vi "ao_ai_dmm_amp_test.vi"() -> ()   [LabVIEW 2020]
uses:
  Realization/PIPX40 Matrix/PIPX40 Matrix.lvclass
  Realization/NI Analog Input/NI Analog Input.lvclass
  Realization/NI DAQmx Base/TypeDefs/Channel Config.ctl
  Realization/NI Analog Output/TypeDefs/Timing Config.ctl
  Realization/NI Analog Output/NI Analog Output.lvclass
  Realization/PIPX40 Relay/PIPX40 Relay.lvclass
  Realization/NI DMM/NI DMM.lvclass
  Realization/PI650 VoltageAmp/PI650 VoltageAmp.lvclass
  Realization/PI650 VoltageAmp/TypeDefs/Channel gain.ctl
  Realization/PI650 VoltageAmp/TypeDefs/Channel DC offset.ctl
  Realization/NI DMM/TypeDefs/DMM waveform settings.ctl
  <instrlib>/niDMM/nidmm.llb/niDMM Waveform Function.ctl
  <instrlib>/niDMM/nidmm.llb/niDMM Function.ctl
panel:
  out "Amp Info":variant
  out "DMM":waveform(dbl)(graph)
  out "DMM Info":variant
  out "AI":waveform(dbl)[](graph)
  out "relay info":variant
  out "AO Info":variant
  out "AI infos":variant[](array[variant])
  out "Mx infos":variant[](array[variant])
  out "error out":errorcluster
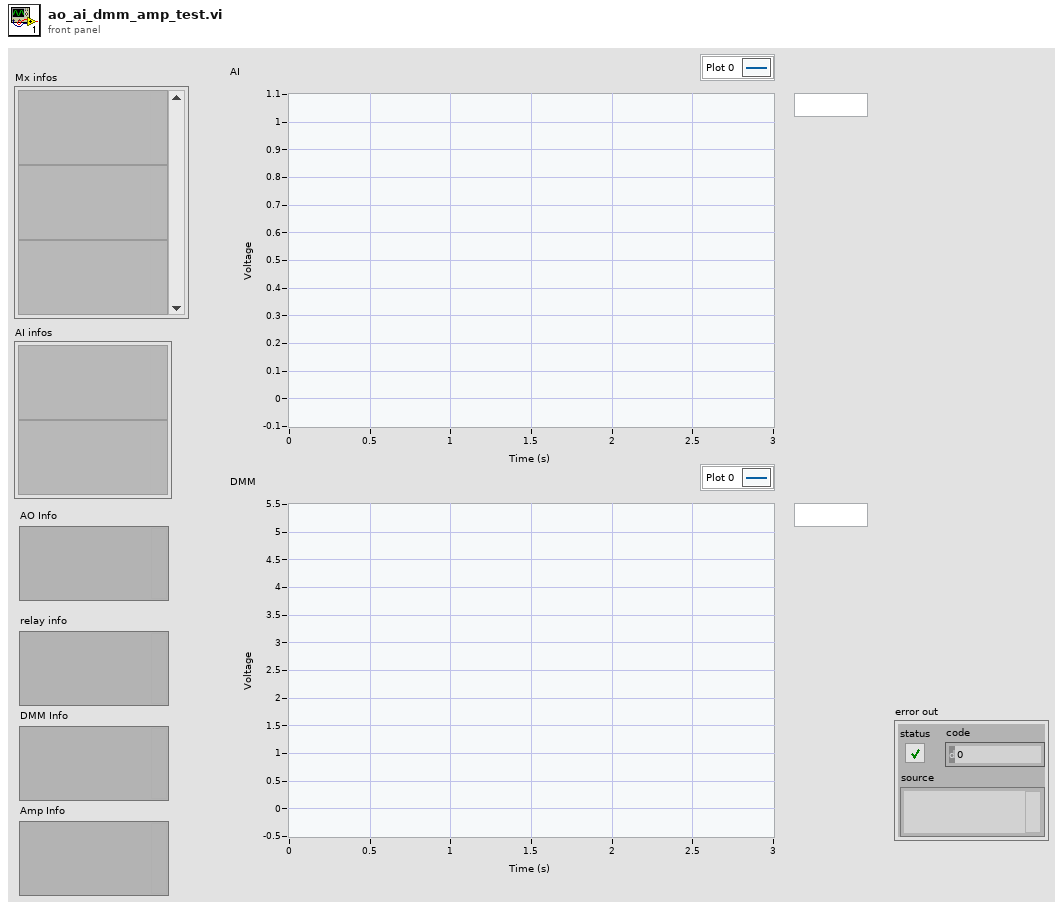
[diagram p1: front panel]
types:
  T1 = typedef "Channel gain.ctl" = cluster{"Channel (CH1)":u32, "Gain (x1)":u32}
  T2 = typedef "Channel Config.ctl" = cluster{"channels":string, "maximum value":dbl, "minimum value":dbl, "output terminal configuration":i32, "units":i32}
  T3 = map{string, refnum<class "NI Analog Input.lvclass">}
  T4 = map{string, refnum<class "PIPX40 Matrix.lvclass">}
  T5 = typedef "Timing Config.ctl" = cluster{"sample mode":i32, "samples per channel":i32, "rate":dbl, "source":string, "active edge":i32}
  T6 = typedef "Rendezvous RefNum" = refnum<k1>
  T7 = typedef "Channel DC offset.ctl" = cluster{"Channel (CH1)":u32, "Offset (128)":u32}
  T8 = typedef "niDMM Function.ctl" = enum16{"DC Volts", "AC Volts", "DC Current", "AC Current", "2-wire Resistance", "4-wire Resistance", "Diode", "Frequency", "Period", "AC Volts DC Coupled", "Capacitance", "Inductance", "Temperature"}
  T9 = cluster{"Function":T8, "Resolution":dbl, "Range":dbl}
  T10 = typedef "DMM waveform settings.ctl" = cluster{"Waveform Points":i32, "Function":T11, "Rate":dbl, "Range":dbl, "Settle Time":dbl}
  T11 = typedef "niDMM Waveform Function.ctl" = i32
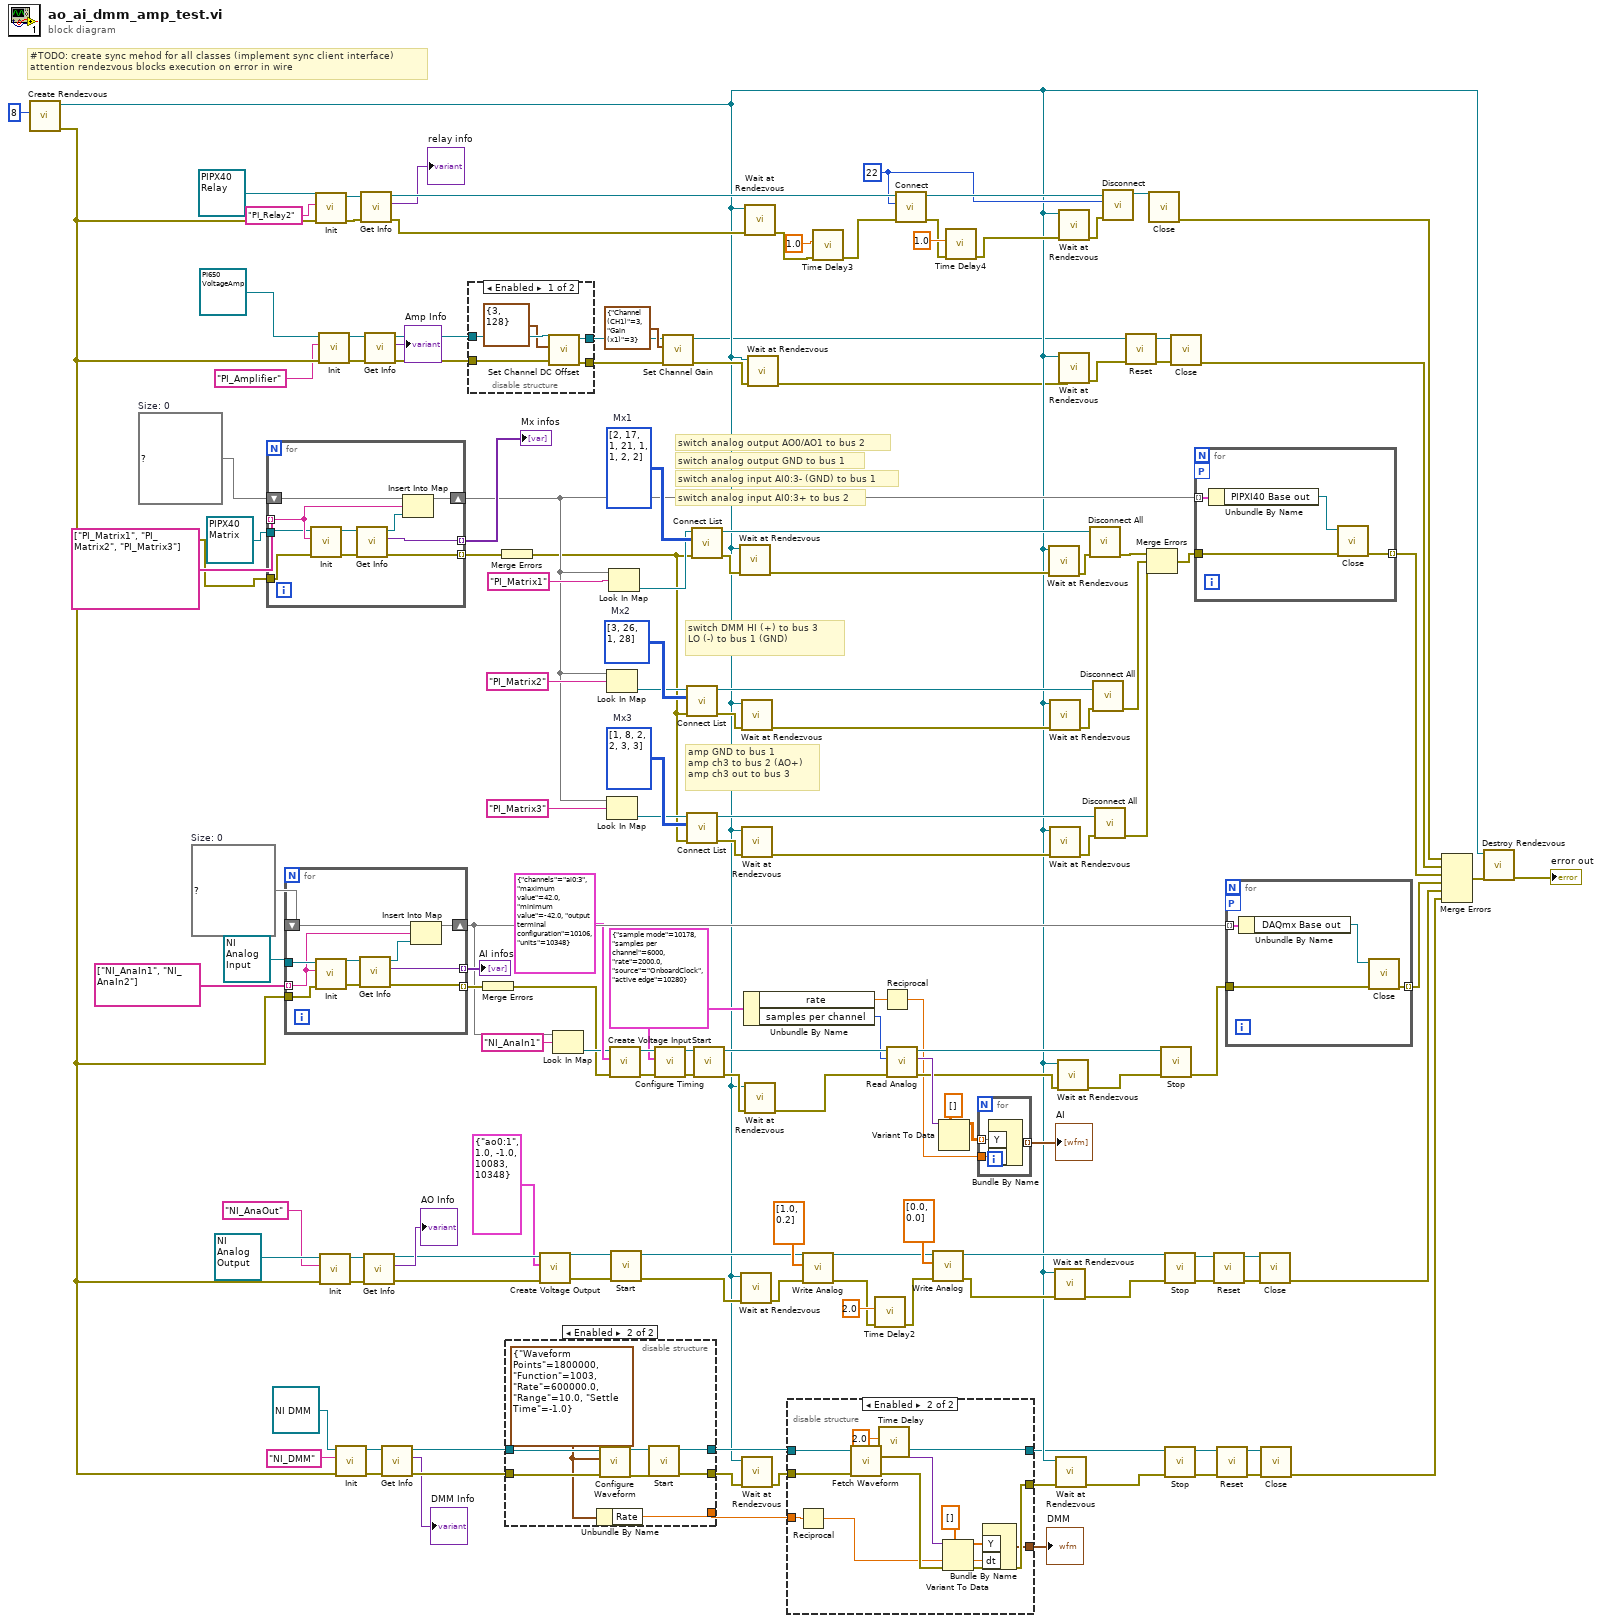
[diagram p0: block diagram]
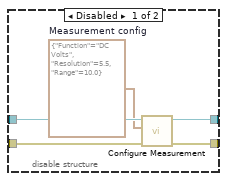
[diagram p3: hidden frame]
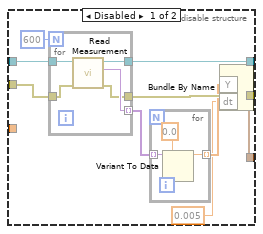
[diagram p4: hidden frame]
diagram:
  w18 = i32[][] [[1, 8], [2, 2], [3, 3]]  # Mx3
  w69 = 22
  w120 = T3 {}  # Size: 0
  w126 = T4 {}  # Size: 0
  w48 = T5 {"sample mode"=10178, "samples per channel"=6000, "rate"=2000.0, "source"="OnboardClock", "active edge"=10280}
  w144 = i32[][] [[3, 26], [1, 28]]  # Mx2
  w146 = i32[][] [[2, 17], [1, 21], [1, 1], [2, 2]]  # Mx1
  # "amp GND to bus 1\namp ch3 to bus 2 (AO+) \namp ch3 out to bus 3"
  # "switch analog input AI0:3+ to bus 2"
  # "switch analog input AI0:3- (GND) to bus 1"
  # "switch analog output GND to bus 1"
  # "switch analog output AO0/AO1 to bus 2"
  # "switch DMM HI (+) to bus 3 \nLO (-) to bus 1 (GND)"
  # "#TODO: create sync mehod for all classes (implement sync client interface)\nattention rendezvous blocks execution on error in wire"
  n1 = call <vilib>:"Create Rendezvous.vi"("size (2)"=8) -> ("error out"=w37:errorcluster, "rendezvous"=w10:T6)  [unwired: 4 in, 1 out]
  n2 = for {
    tunnel: string[] ["PI_Matrix1", "PI_Matrix2", "PI_Matrix3"] -> [w157] mode=indexing
    tunnel: [w160] -> w150 mode=indexing
    tunnel: [w159] -> w148 mode=indexing
    shift-right: [w158] -> w12
    shift-left: w126 -> [w155]
    tunnel: refnum<class "PIPX40 Matrix.lvclass"> refnum ("PIPXI40 Matrix in") -> [w153]
    tunnel: w37 -> [w152]
    n3 = call-dynamic "Init.vi"("error in (no error)"=w152, "Params"=w157, "PIPXI40 Base in"=w153) -> ("error out"=w161:errorcluster, "PIPXI40 Base out"=w156:refnum<class "PIPX40 Matrix.lvclass">)  [unwired: 7 in]
    n4 = call-dynamic "Get Info.vi"("error in (no error)"=w161, "PIPXI40 Base in"=w156) -> ("error out"=w160:errorcluster, "Info"=w159:variant, "PIPXI40 Base out"=w154:refnum<class "PIPX40 Matrix.lvclass">)  [unwired: 7 in]
    n5 = Insert Into Map(map in=w155, key=w157, value=w154) -> (map out=w158:T4)  [unwired: 2 out]
  }
  "Mx infos" <- w148
  n6 = for {
    tunnel: string[] ["NI_AnaIn1", "NI_AnaIn2"] -> [w163] mode=indexing
    shift-right: [w171] -> w134
    shift-left: w120 -> [w170]
    tunnel: refnum<class "NI Analog Input.lvclass"> refnum ("NI Analog Input in") -> [w169]
    tunnel: [w165] -> w137 mode=indexing
    tunnel: [w164] -> w136 mode=indexing
    tunnel: w37 -> [w162]
    n7 = call-dynamic "Init.vi"("error in (no error)"=w162, "Params"=w163, "DAQmx Base in"=w169) -> ("error out"=w167:errorcluster, "DAQmx Base out"=w168:refnum<class "NI Analog Input.lvclass">)  [unwired: 7 in]
    n8 = call-dynamic "Get Info.vi"("error in (no error)"=w167, "DAQmx Base in"=w168) -> ("error out"=w164:errorcluster, "Info"=w165:variant, "DAQmx Base out"=w166:refnum<class "NI Analog Input.lvclass">)  [unwired: 7 in]
    n9 = Insert Into Map(map in=w170, key=w163, value=w166) -> (map out=w171:T3)  [unwired: 2 out]
  }
  "AI infos" <- w137
  n10 = call-dynamic "Init.vi"("error in (no error)"=w37, "Params"="PI_Relay2" ("String"), "PIPXI40 Base in"=refnum<class "PIPX40 Relay.lvclass"> refnum ("Pickering.lvlib:PIPX40 Relay.lvclass")) -> ("error out"=w106:errorcluster, "PIPXI40 Base out"=w103:refnum<class "PIPX40 Relay.lvclass">)  [unwired: 7 in]
  n11 = call-dynamic "Init.vi"("error in (no error)"=w37, "Params"="PI_Amplifier" ("String"), "PI650 VoltageAmp in"=refnum<class "PI650 VoltageAmp.lvclass"> refnum) -> ("error out"=w28:errorcluster, "PI650 VoltageAmp out"=w29:refnum<class "PI650 VoltageAmp.lvclass">)  [unwired: 7 in]
  n12 = call-dynamic "Init.vi"("error in (no error)"=w37, "Params"="NI_AnaOut" ("String"), "DAQmx Base in"=refnum<class "NI Analog Output.lvclass"> refnum ("NI DAQmx.lvlib:NI Analog Output.lvclass")) -> ("error out"=w118:errorcluster, "DAQmx Base out"=w119:refnum<class "NI Analog Output.lvclass">)  [unwired: 7 in]
  n13 = call-dynamic "Init.vi"("error in (no error)"=w37, "Params"="NI_DMM", "NI DMM in"=refnum<class "NI DMM.lvclass"> refnum) -> ("error out"=w59:errorcluster, "NI DMM out"=w60:refnum<class "NI DMM.lvclass">)  [unwired: 7 in]
  n14 = call-dynamic "Get Info.vi"("error in (no error)"=w106, "PIPXI40 Base in"=w103) -> ("error out"=w98:errorcluster, "Info"=→"relay info":variant, "PIPXI40 Base out"=w102:refnum<class "PIPX40 Relay.lvclass">)  [unwired: 7 in]
  n15 = call-dynamic "Get Info.vi"("error in (no error)"=w118, "DAQmx Base in"=w119) -> ("error out"=w114:errorcluster, "Info"=→"AO Info":variant, "DAQmx Base out"=w115:refnum<class "NI Analog Output.lvclass">)  [unwired: 7 in]
  n16 = call-dynamic "Get Info.vi"("error in (no error)"=w28, "PI650 VoltageAmp in"=w29) -> ("error out"=w27:errorcluster, "Info"=→"Amp Info":variant, "PI650 VoltageAmp out"=w30:refnum<class "PI650 VoltageAmp.lvclass">)  [unwired: 7 in]
  n17 = call-dynamic "Get Info.vi"("error in (no error)"=w59, "NI DMM in"=w60) -> ("error out"=w57:errorcluster, "Info"=→"DMM Info":variant, "NI DMM out"=w58:refnum<class "NI DMM.lvclass">)  [unwired: 7 in]
  n18 = disable-structure shown="Enabled" {
    disable-tunnel: w30 -> [w176 w178]
    disable-tunnel: w27 -> [w175 w177]
    disable-tunnel: [w173 w178] -> w21
    disable-tunnel: [w172 w177] -> w20
    frame Enabled {
      n19 = call-dynamic "Set Channel DC Offset.vi"("error in (no error)"=w175, "Params"=T7 {"Channel (CH1)"=3, "Offset (128)"=128}, "PI650 VoltageAmp in"=w176) -> ("error out"=w172:errorcluster, "PI650 VoltageAmp out"=w173:refnum<class "PI650 VoltageAmp.lvclass">)  [unwired: 7 in]
    }
    frame Disabled {
    }
  }
  n20 = Merge Errors(w136) -> (w95:errorcluster)
  n21 = Merge Errors(w150) -> (w11:errorcluster)
  n22 = disable-structure shown="Enabled" {
    disable-tunnel: w58 -> [w183 w191]
    disable-tunnel: w57 -> [w182 w190]
    disable-tunnel: [w180 w187] -> w55
    disable-tunnel: [w179 w186] -> w54
    disable-tunnel: [_ w184] -> w40
    frame Disabled {
      w181 = T9 {"Function"=enum."DC Volts", "Resolution"=5.5, "Range"=10.0}  # Measurement config
      n23 = call-dynamic "Configure Measurement.vi"("error in (no error)"=w182, "Params"=w181, "NI DMM in"=w183) -> ("error out"=w180:errorcluster, "NI DMM out"=w179:refnum<class "NI DMM.lvclass">)  [unwired: 7 in]
    }
    frame Enabled {
      w185 = T10 {"Waveform Points"=1800000, "Function"=1003, "Rate"=600000.0, "Range"=10.0, "Settle Time"=-1.0}
      n24 = Unbundle By Name(w185) -> ("Rate"=w184:dbl)
      n25 = call-dynamic "Configure Waveform.vi"("error in (no error)"=w190, "Params"=w185, "NI DMM in"=w191) -> ("error out"=w188:errorcluster, "NI DMM out"=w189:refnum<class "NI DMM.lvclass">)  [unwired: 7 in]
      n26 = call-dynamic "Start.vi"("error in (no error)"=w188, "DMM in"=w189) -> ("error out"=w187:errorcluster, "DMM out"=w186:refnum<class "NI DMM.lvclass">)  [unwired: 8 in]
    }
  }
  n27 = call-dynamic "Create Voltage Output.vi"("error in (no error)"=w114, "Params"=T2 {"channels"="ao0:1", "maximum value"=1.0, "minimum value"=-1.0, "output terminal configuration"=10083, "units"=10348} ("Channel Config"), "NI Analog Output in"=w115) -> ("error out"=w92:errorcluster, "NI Analog Output out"=w91:refnum<class "NI Analog Output.lvclass">)  [unwired: 7 in]
  n28 = Look In Map(map=w134, key="NI_AnaIn1") -> (value=w123:refnum<class "NI Analog Input.lvclass">)  [unwired: 1 in, 1 out]
  n29 = Look In Map(map=w12, key="PI_Matrix2" ("String")) -> (value=w128:refnum<class "PIPX40 Matrix.lvclass">)  [unwired: 1 in, 1 out]
  n30 = Look In Map(map=w12, key="PI_Matrix3" ("String")) -> (value=w16:refnum<class "PIPX40 Matrix.lvclass">)  [unwired: 1 in, 1 out]
  n31 = Look In Map(map=w12, key="PI_Matrix1" ("String")) -> (value=w132:refnum<class "PIPX40 Matrix.lvclass">)  [unwired: 1 in, 1 out]
  n32 = call-dynamic "Create Voltage Input.vi"("error in (no error)"=w95, "Params"=T2 {"channels"="ai0:3", "maximum value"=42.0, "minimum value"=-42.0, "output terminal configuration"=10106, "units"=10348} ("Channel Config"), "NI Analog Input in"=w123) -> ("error out"=w130:errorcluster, "NI Analog Input out"=w122:refnum<class "NI Analog Input.lvclass">)  [unwired: 7 in]
  n33 = call-dynamic "Start.vi"("error in (no error)"=w92, "NI DAQmx Base in"=w91) -> ("error out"=w89:errorcluster, "NI DAQmx Base out"=w90:refnum<class "NI Analog Output.lvclass">)  [unwired: 8 in]
  n34 = call-dynamic "Configure Timing.vi"("error in (no error)"=w130, "Params"=w48, "NI DAQmx Base in"=w122) -> ("error out"=w87:errorcluster, "NI DAQmx Base out"=w86:refnum<class "NI Analog Input.lvclass">)  [unwired: 7 in]
  n35 = call-dynamic "Set Channel Gain.vi"("error in (no error)"=w20, "Params"=T1 {"Channel (CH1)"=3, "Gain (x1)"=3} ("Channel gain"), "PI650 VoltageAmp in"=w21) -> ("error out"=w36:errorcluster, "PI650 VoltageAmp out"=w6:refnum<class "PI650 VoltageAmp.lvclass">)  [unwired: 7 in]
  n36 = call-dynamic "Connect List.vi"("error in (no error)"=w11, "Params"=w144, "PIPXI40 Matrix in"=w128) -> ("error out"=w94:errorcluster, "PIPXI40 Matrix out"=w142:refnum<class "PIPX40 Matrix.lvclass">)  [unwired: 7 in]
  n37 = call-dynamic "Connect List.vi"("error in (no error)"=w11, "Params"=w18, "PIPXI40 Matrix in"=w16) -> ("error out"=w15:errorcluster, "PIPXI40 Matrix out"=w17:refnum<class "PIPX40 Matrix.lvclass">)  [unwired: 7 in]
  n38 = call-dynamic "Connect List.vi"("error in (no error)"=w11, "Params"=w146, "PIPXI40 Matrix in"=w132) -> ("error out"=w93:errorcluster, "PIPXI40 Matrix out"=w143:refnum<class "PIPX40 Matrix.lvclass">)  [unwired: 7 in]
  n39 = call-dynamic "Start.vi"("error in (no error)"=w87, "NI DAQmx Base in"=w86) -> ("error out"=w84:errorcluster, "NI DAQmx Base out"=w85:refnum<class "NI Analog Input.lvclass">)  [unwired: 8 in]
  n40 = call <vilib>:"Wait at Rendezvous.vi"("error in (no error)"=w93, "rendezvous"=w10) -> ("error out"=w79:errorcluster)  [unwired: 3 in, 2 out]
  n41 = call <vilib>:"Wait at Rendezvous.vi"("error in (no error)"=w89, "rendezvous"=w10) -> ("error out"=w88:errorcluster)  [unwired: 3 in, 2 out]
  n42 = call <vilib>:"Wait at Rendezvous.vi"("error in (no error)"=w94, "rendezvous"=w10) -> ("error out"=w75:errorcluster)  [unwired: 3 in, 2 out]
  n43 = call <vilib>:"Wait at Rendezvous.vi"("error in (no error)"=w15, "rendezvous"=w10) -> ("error out"=w13:errorcluster)  [unwired: 3 in, 2 out]
  n44 = call <vilib>:"Wait at Rendezvous.vi"("error in (no error)"=w55, "rendezvous"=w10) -> ("error out"=w46:errorcluster)  [unwired: 3 in, 2 out]
  n45 = Unbundle By Name(w48) -> ("rate"=w45:dbl, "samples per channel"=w47:i32)
  n46 = call <vilib>:"Wait at Rendezvous.vi"("error in (no error)"=w98, "rendezvous"=w10) -> ("error out"=w8:errorcluster)  [unwired: 3 in, 2 out]
  n47 = call <vilib>:"Wait at Rendezvous.vi"("error in (no error)"=w84, "rendezvous"=w10) -> ("error out"=w83:errorcluster)  [unwired: 3 in, 2 out]
  n48 = call <vilib>:"Wait at Rendezvous.vi"("error in (no error)"=w36, "rendezvous"=w10) -> ("error out"=w5:errorcluster)  [unwired: 3 in, 2 out]
  n49 = disable-structure shown="Enabled" {
    disable-tunnel: w54 -> [w200 w212]
    disable-tunnel: [w199 w217] -> w4
    disable-tunnel: [w197 w218] -> w49
    disable-tunnel: w46 -> [w196 w211]
    disable-tunnel: [w192 w214] -> w41
    disable-tunnel: w40 -> [_ w210]
    frame Disabled {
      n50 = for {
        N: 600 -> [_]
        tunnel: [w206] -> w198 mode=indexing
        tunnel: w200 -> [w208]
        tunnel: [w207] -> w199
        tunnel: w196 -> [w204]
        tunnel: [w205] -> w197
        n51 = call-dynamic "Read Measurement.vi"("error in (no error)"=w204, "DMM in"=w208) -> ("error out"=w205:errorcluster, "Data"=w206:variant, "DMM out"=w207:refnum<class "NI DMM.lvclass">)  [unwired: 7 in]
      }
      n52 = for {
        tunnel: w198 -> [w203] mode=indexing
        tunnel: [w201] -> w194 mode=indexing
        n53 = Variant To Data(type=0.0, Variant=w203) -> (data=w201:dbl)  [unwired: 1 in, 1 out]
      }
      n54 = Bundle By Name("Y"=w194, "dt"=0.005) -> (w192:waveform(dbl))  [unwired: 1 in]
    }
    frame Enabled {
      n55 = Reciprocal(x=w210) -> (1/x=w209:dbl)
      n56 = call-dynamic "Fetch Waveform.vi"("error in (no error)"=w211, "NI DMM in"=w212) -> ("error out"=w219:errorcluster, "Data"=w216:variant, "NI DMM out"=w217:refnum<class "NI DMM.lvclass">)  [unwired: 7 in]
      n57 = Variant To Data(error in=w219, type=dbl[] [], Variant=w216) -> (data=w213:dbl[], error out=w218:errorcluster)
      n58 = Bundle By Name("Y"=w213, "dt"=w209) -> (w214:waveform(dbl))  [unwired: 1 in]
    }
  }
  "DMM" <- w41
  n59 = call-dynamic "Write Analog.vi"("error in (no error)"=w88, "Params"=dbl[] [1.0, 0.2] ("element"), "NI Analog Output in"=w90) -> ("error out"=w33:errorcluster, "NI Analog Output out"=w65:refnum<class "NI Analog Output.lvclass">)  [unwired: 7 in]
  n60 = call "Time Delay3"("error in (no error)"=w8, "Delay Time (s)"=1.0) -> ("error out"=w7:errorcluster)  [unwired: 9 in]
  n61 = call "Time Delay2"("error in (no error)"=w33, "Delay Time (s)"=2.0) -> ("error out"=w32:errorcluster)  [unwired: 9 in]
  n62 = call "Time Delay"("Delay Time (s)"=2.0) -> ()  [unwired: 10 in, 1 out]
  n63 = Reciprocal(x=w45) -> (1/x=w42:dbl)
  n64 = call-dynamic "Read Analog.vi"("error in (no error)"=w83, "Params"=w47, "NI Analog Input in"=w85) -> ("error out"=w74:errorcluster, "Data"=w125:variant, "NI Analog Input out"=w77:refnum<class "NI Analog Input.lvclass">)  [unwired: 6 in]
  n65 = call-dynamic "Connect.vi"("error in (no error)"=w7, "Params"=w69, "Switching in"=w102) -> ("error out"=w81:errorcluster, "Switching out"=w71:refnum<class "PIPX40 Relay.lvclass">)  [unwired: 7 in]
  n66 = call-dynamic "Write Analog.vi"("error in (no error)"=w32, "Params"=dbl[] [0.0, 0.0] ("element"), "NI Analog Output in"=w65) -> ("error out"=w64:errorcluster, "NI Analog Output out"=w63:refnum<class "NI Analog Output.lvclass">)  [unwired: 7 in]
  n67 = Variant To Data(type=dbl[][] [], Variant=w125) -> (data=w44:dbl[][])  [unwired: 1 in, 1 out]
  n68 = call "Time Delay4"("error in (no error)"=w81, "Delay Time (s)"=1.0) -> ("error out"=w67:errorcluster)  [unwired: 9 in]
  n69 = for {
    tunnel: w44 -> [w222] mode=indexing
    tunnel: [w221] -> w43 mode=indexing
    tunnel: w42 -> [w220]
    n70 = Bundle By Name("Y"=w222, "dt"=w220) -> (w221:waveform(dbl))  [unwired: 1 in]
  }
  "AI" <- w43
  n71 = call <vilib>:"Wait at Rendezvous.vi"("error in (no error)"=w79, "rendezvous"=w10) -> ("error out"=w78:errorcluster)  [unwired: 3 in, 2 out]
  n72 = call <vilib>:"Wait at Rendezvous.vi"("error in (no error)"=w75, "rendezvous"=w10) -> ("error out"=w76:errorcluster)  [unwired: 3 in, 2 out]
  n73 = call <vilib>:"Wait at Rendezvous.vi"("error in (no error)"=w13, "rendezvous"=w10) -> ("error out"=w14:errorcluster)  [unwired: 3 in, 2 out]
  n74 = call <vilib>:"Wait at Rendezvous.vi"("error in (no error)"=w64, "rendezvous"=w10) -> ("error out"=w72:errorcluster)  [unwired: 3 in, 2 out]
  n75 = call <vilib>:"Wait at Rendezvous.vi"("error in (no error)"=w49, "rendezvous"=w10) -> ("error out"=w3:errorcluster)  [unwired: 3 in, 2 out]
  n76 = call <vilib>:"Wait at Rendezvous.vi"("error in (no error)"=w74, "rendezvous"=w10) -> ("error out"=w73:errorcluster)  [unwired: 3 in, 2 out]
  n77 = call <vilib>:"Wait at Rendezvous.vi"("error in (no error)"=w67, "rendezvous"=w10) -> ("error out"=w68:errorcluster)  [unwired: 3 in, 2 out]
  n78 = call <vilib>:"Wait at Rendezvous.vi"("error in (no error)"=w5, "rendezvous"=w10) -> ("error out"=w35:errorcluster)  [unwired: 3 in, 2 out]
  n79 = call-dynamic "Disconnect All.vi"("error in (no error)"=w78, "PIPXI40 Matrix in"=w143) -> ("error out"=w140:errorcluster)  [unwired: 8 in, 1 out]
  n80 = call-dynamic "Disconnect All.vi"("error in (no error)"=w76, "PIPXI40 Matrix in"=w142) -> ("error out"=w141:errorcluster)  [unwired: 8 in, 1 out]
  n81 = call-dynamic "Disconnect All.vi"("error in (no error)"=w14, "PIPXI40 Matrix in"=w17) -> ("error out"=w9:errorcluster)  [unwired: 8 in, 1 out]
  n82 = call-dynamic "Disconnect.vi"("error in (no error)"=w68, "Params"=w69, "Switching in"=w71) -> ("Switching out"=w70:refnum<class "PIPX40 Relay.lvclass">)  [unwired: 7 in, 1 out]
  n83 = call-dynamic "Reset.vi"("error in (no error)"=w35, "PI650 VoltageAmp in"=w6) -> ("error out"=w24:errorcluster, "PI650 VoltageAmp out"=w23:refnum<class "PI650 VoltageAmp.lvclass">)  [unwired: 8 in]
  n84 = Merge Errors(w140, w141, w9) -> (w139:errorcluster)
  n85 = call-dynamic "Close.vi"("PIPXI40 Base in"=w70) -> ("error out"=w39:errorcluster)  [unwired: 9 in, 1 out]
  n86 = call-dynamic "Stop.vi"("error in (no error)"=w73, "NI DAQmx Base in"=w77) -> ("error out"=w96:errorcluster)  [unwired: 8 in, 1 out]
  n87 = call-dynamic "Stop.vi"("error in (no error)"=w72, "NI DAQmx Base in"=w63) -> ("error out"=w112:errorcluster, "NI DAQmx Base out"=w111:refnum<class "NI Analog Output.lvclass">)  [unwired: 8 in]
  n88 = call-dynamic "Stop.vi"("error in (no error)"=w3, "NI DMM in"=w4) -> ("error out"=w1:errorcluster, "NI DMM out"=w2:refnum<class "NI DMM.lvclass">)  [unwired: 8 in]
  n89 = call-dynamic "Close.vi"("error in (no error)"=w24, "PI650 VoltageAmp in"=w23) -> ("error out"=w38:errorcluster)  [unwired: 8 in, 1 out]
  n90 = for {
    tunnel: w139 -> [w225]
    tunnel: [w226] -> w149 mode=indexing
    workers-P: _ -> [_]
    tunnel: w12 -> [w224] mode=indexing
    n91 = Unbundle By Name(w224) -> ("PIPXI40 Base out"=w223:refnum<class "PIPX40 Matrix.lvclass">)
    n92 = call-dynamic "Close.vi"("error in (no error)"=w225, "PIPXI40 Base in"=w223) -> ("error out"=w226:errorcluster)  [unwired: 8 in, 1 out]
  }
  n93 = call-dynamic "Reset.vi"("error in (no error)"=w112, "DAQmx Base in"=w111) -> ("error out"=w110:errorcluster, "DAQmx Base out"=w109:refnum<class "NI Analog Output.lvclass">)  [unwired: 8 in]
  n94 = call-dynamic "Reset.vi"("error in (no error)"=w1, "NI DMM in"=w2) -> ("error out"=w52:errorcluster, "NI DMM out"=w53:refnum<class "NI DMM.lvclass">)  [unwired: 8 in]
  n95 = for {
    tunnel: w96 -> [w229]
    tunnel: [w230] -> w135 mode=indexing
    workers-P: _ -> [_]
    tunnel: w134 -> [w228] mode=indexing
    n96 = Unbundle By Name(w228) -> ("DAQmx Base out"=w227:refnum<class "NI Analog Input.lvclass">)
    n97 = call-dynamic "Close.vi"("error in (no error)"=w229, "DAQmx Base in"=w227) -> ("error out"=w230:errorcluster)  [unwired: 8 in, 1 out]
  }
  n98 = call-dynamic "Close.vi"("error in (no error)"=w110, "DAQmx Base in"=w109) -> ("error out"=w108:errorcluster)  [unwired: 8 in, 1 out]
  n99 = call-dynamic "Close.vi"("error in (no error)"=w52, "NI DMM in"=w53) -> ("error out"=w51:errorcluster)  [unwired: 8 in, 1 out]
  n100 = Merge Errors(w39, w38, w149, w135, w108, w51) -> (w100:errorcluster)
  n101 = call <vilib>:"Destroy Rendezvous.vi"("error in (no error)"=w100, "rendezvous"=w10) -> ("error out"=→"error out":errorcluster)  [unwired: 4 in, 1 out]
